vi "Read Model Number.vi"(8 "error in (no error)":errorcluster, 11 "String":string="0.0.0.0") -> (0 "error out":errorcluster, 3 "Target Info":T1)   [LabVIEW 2015]
uses:
  <vilib>/nisyscfg/Close (System).vi
  <vilib>/nisyscfg/nisyscfg.lvlib
  <resource>/objmgr/nisysapi.rc
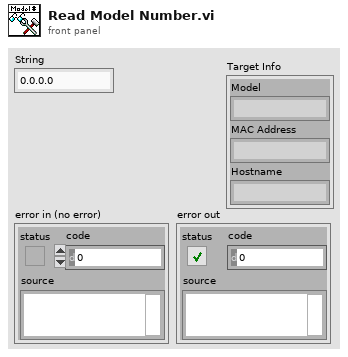
[diagram p1: front panel]
types:
  T1 = cluster{"Model":string, "MAC Address":string, "Hostname":string}
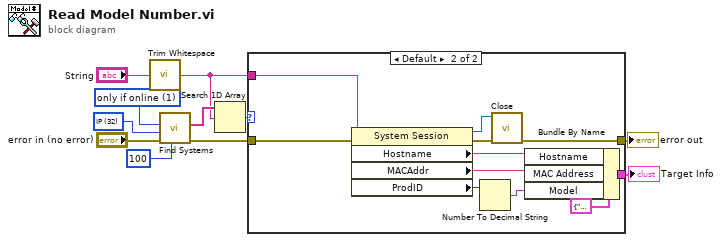
[diagram p0: block diagram]
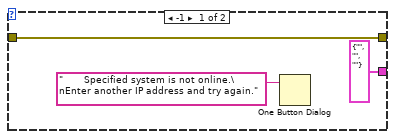
[diagram p2: hidden frame]
diagram:
  w5 = u32 1 items=["none"=0, "only if online"=1, "all"=3] ("Include Cached Results (all)")
  w6 = u32 32 items=["Hostname"=16, "Hostname (IP)"=18, "Hostname (MAC)"=19, "IP"=32, "IP (Hostname)"=33, "IP (MAC)"=35, "MAC"=48, "MAC (Hostname)"=49, "MAC (IP)"=50] ("Output (Hostname and IP)")
  n1 = call <vilib>:"Trim Whitespace.vi"("string"="String") -> ("trimmed string"=w1:string)  [unwired: 1 in]
  n2 = call <vilib>:"Find Systems.vi"("Timeout (4000 ms)"=u32 100, "error in (no error)"="error in (no error)", "Output (Hostname and IP)"=w6, "Include Cached Results (all)"=w5) -> ("error out"=w8:errorcluster, "Detected Systems"=w4:string[])  [unwired: 5 in, 1 out]
  n3 = Search 1D Array(1D array=w4, element=w1) -> (index of element=w3:i32)  [unwired: 1 in]
  n4 = case shown="Default" w3 {
    tunnel: [w14 w23] -> w11
    tunnel: [T1 {"Model"="", "MAC Address"="", "Hostname"=""} ("input cluster") w17] -> w10
    tunnel: w8 -> [w14 w16]
    tunnel: w1 -> [_ w15]
    frame -1 {
      n5 = One Button Dialog(message="       Specified system is not online.\nEnter another IP address and try again.") -> ()  [unwired: 1 in, 1 out]
    }
    frame Default {
      n6 = property class="System Session"(reference=w15, error in=w16) -> (reference out=w25:refnum<k21>, error out=w24:errorcluster, "Hostname"=w18:string, "MACAddr"=w21:string, "ProdID"=w20:i32)
      n7 = Number To Decimal String(number=w20) -> (decimal integer string=w19:string)  [unwired: 1 in]
      n8 = call-poly <vilib>:"Close.vi"("error in (no error)"=w24, "Session in"=w25) -> ("error out"=w23:errorcluster)  [unwired: 9 in]
      n9 = Bundle By Name(cluster=T1 {"Model"="", "MAC Address"="", "Hostname"=""} ("input cluster"), "Hostname"=w18, "MAC Address"=w21, "Model"=w19) -> (w17:T1)
    }
  }
  "error out" <- w11
  "Target Info" <- w10
